vi "9219_RtdRangeString.vi"(8 "_Degree Range":u8(ring) items=["Raw units", "Degrees Kelvin", "Degrees Celsius", "Degrees Fahrenheit", "Degrees Rankine"], 9 "_Range":u8, 11 "RTD Type":u8(ring) items=["TCR3851"=1, "TCR3750"=2, "TCR3916"=3, "TCR3920"=4, "TCR3911"=5, "TCR3928"=6, "Custom"=0]) -> (2 "_RTD String":string)   [LabVIEW 2020, in "Modules.lvlib" / "9219.lvclass"]
uses:
  9219.lvclass
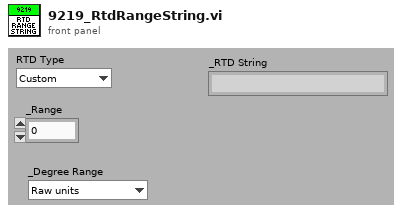
[diagram p1: front panel]
types:
  T1 = typedef "LVStringsAndValuesArrayTypeDef_U8.ctl" = cluster{"String":string, "Value":u8}[]
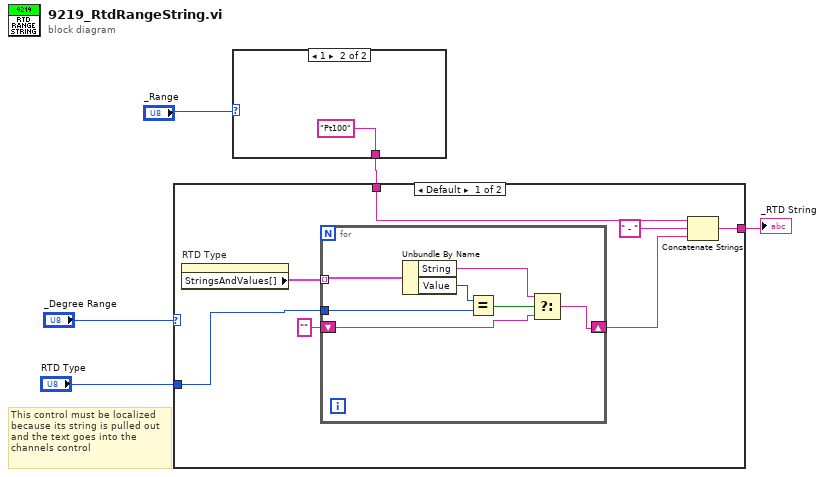
[diagram p0: block diagram]
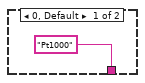
[diagram p3: hidden frame]
diagram:
  # "This control must be localized\nbecause its string is pulled out\nand the text goes into the \nchannels control"
  n1 = case shown="1" "_Range" {
    tunnel: ["Pt1000" ("String") "Pt100" ("String")] -> w5
    frame 0, Default {
    }
    frame 1 {
    }
  }
  n2 = case shown="Default" "_Degree Range" {
    tunnel: w5 -> [w12 w22]
    tunnel: [w11 w22] -> w4
    tunnel: "RTD Type" -> [w8 _]
    frame Default {
      n3 = property on="RTD Type" class="Ring (strict)"() -> ("StringsAndValues[]"=w14:T1)  [unwired: 2 in, 2 out]
      n4 = for {
        tunnel: w14 -> [w21] mode=indexing
        tunnel: w8 -> [w19]
        shift-right: [w16] -> w9
        shift-left: "" ("String") -> [w15]
        n5 = Unbundle By Name(w21) -> ("String"=w17:string, "Value"=w20:u8)
        n6 = Equal?(x=w20, y=w19) -> (x = y?=w18:bool)
        n7 = Select(t=w17, s=w18, f=w15) -> (s? t:f=w16:string)
      }
      n8 = Concatenate Strings(w12, " - " ("string"), w9) -> (w11:string)
    }
    frame 0 {
      # "0 - Raw Ohms\n\nNO RTD TYPE"
    }
  }
  "_RTD String" <- w4
